vi "DEMO(读取MAC).vi"() -> ()   [LabVIEW 2012]
uses:
  ManagementClass/ManagementClass.lvclass
panel:
  out "Parameters":string[](array[string])
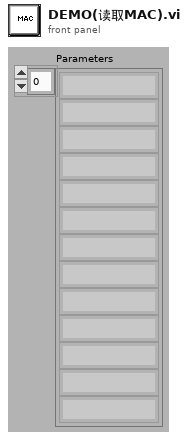
[diagram p1: front panel]
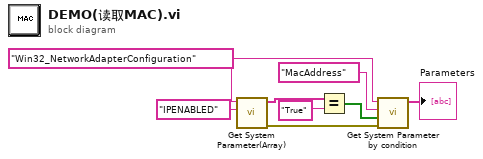
[diagram p0: block diagram]
diagram:
  w4 = "Win32_NetworkAdapterConfiguration" ("path")
  n1 = call "Get System Parameter(Array).vi"("propertyName"="IPENABLED", "path"=w4) -> ("error out"=w5:errorcluster, "Parameters"=w7:string[])  [unwired: 8 in]
  n2 = Equal?(x=w7, y="True") -> (x = y?=w2:bool[])
  n3 = call "Get System Parameter by condition.vi"("error in (no error)"=w5, "Enable"=w2, "propertyName"="MacAddress", "path"=w4) -> ("Parameters"=→"Parameters":string[])  [unwired: 6 in, 1 out]
